vi "SplitPAQsavedPortion.vi"(8 "error in":errorcluster, 9 "split-index":i32, 11 "SaveData in":T1) -> (0 "error out":errorcluster, 2 "SaveData out Day2":T1, 3 "SaveData out Day1":T1)   [LabVIEW 2014, in "DBAL-BIN.lvclass"]
doc: "Split a Database save portion in two halves.\nThe indez input is the point where one day is passed on into another."
uses:
  DBAL-BIN.lvclass
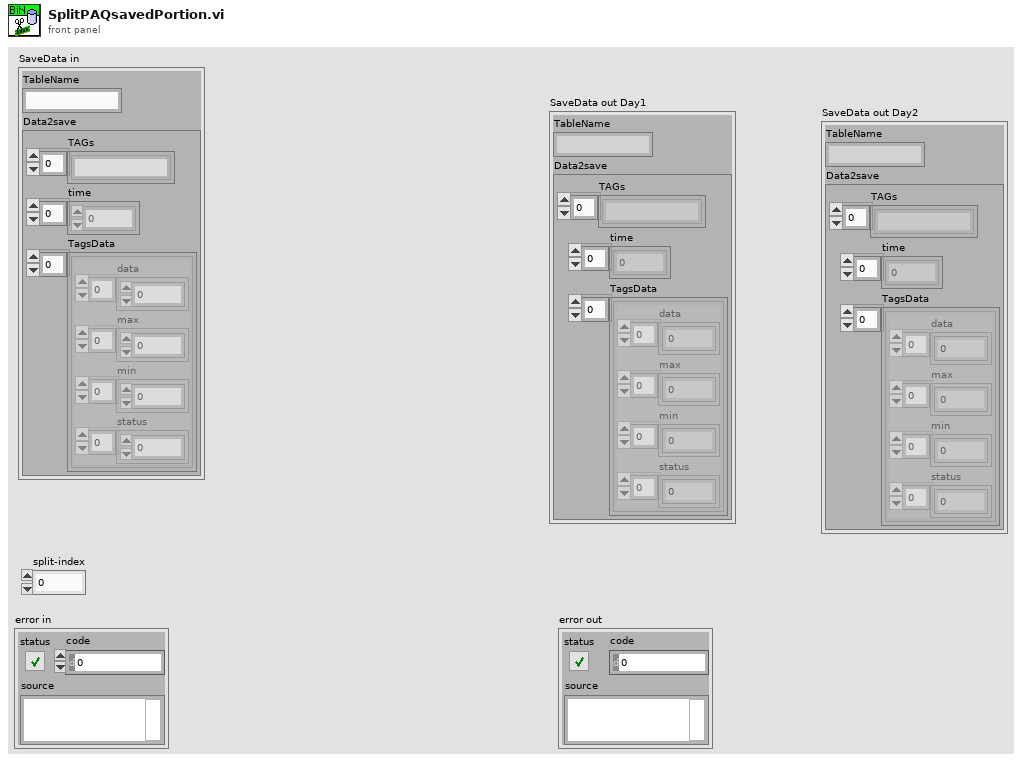
[diagram p1: front panel]
types:
  T1 = cluster{"TableName":string, "Data2save":cluster{"TAGs":string[], "time":dbl[], "TagsData":cluster{"data":dbl[], "max":dbl[], "min":dbl[], "status":u32[]}[]}}
  T2 = cluster{"data":dbl[], "max":dbl[], "min":dbl[], "status":u32[]}[]
  T3 = cluster{"data":dbl[], "max":dbl[], "min":dbl[], "status":u32[]}
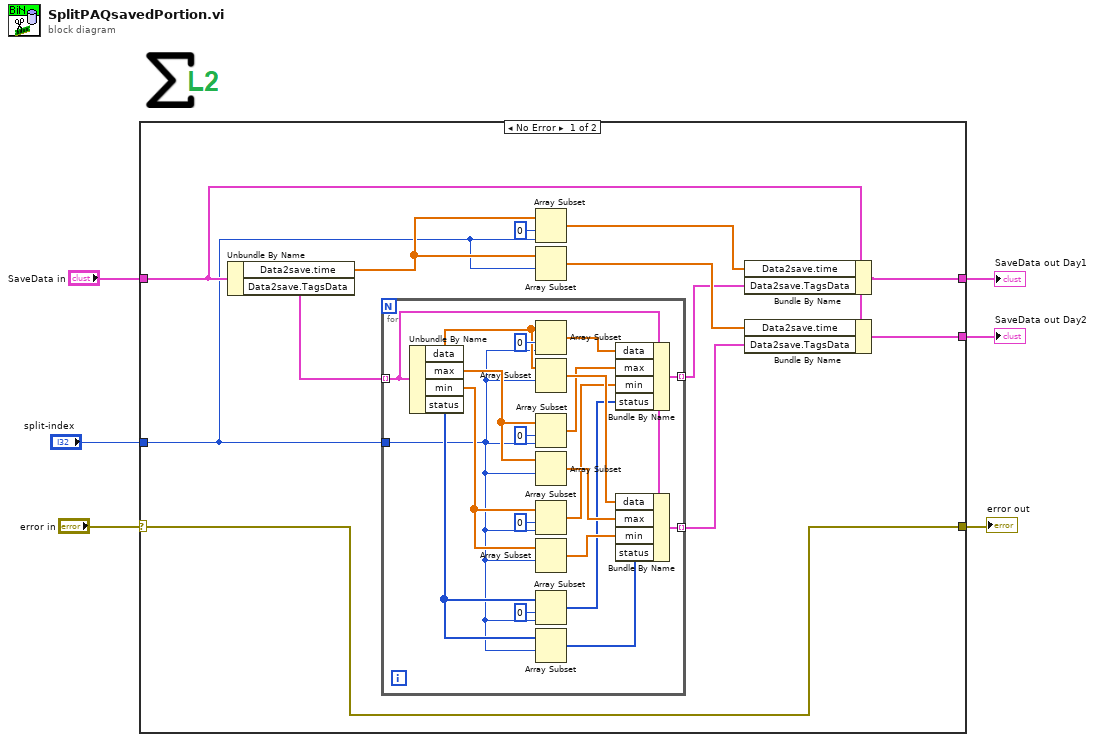
[diagram p0: block diagram]
diagram:
  n1 = case shown="No Error" "error in" {
    selector: "error in" -> [w7 w40]
    tunnel: [w7 w40] -> w6
    tunnel: "SaveData in" -> [w15 w39]
    tunnel: [w17 w39] -> w3
    tunnel: [w16 w39] -> w2
    tunnel: "split-index" -> [w10 _]
    frame No Error {
      n2 = Unbundle By Name(w15) -> ("Data2save.time"=w14:dbl[], "Data2save.TagsData"=w18:T2)
      n3 = for {
        tunnel: w18 -> [w19] mode=indexing
        tunnel: w10 -> [w30]
        tunnel: [w21] -> w9 mode=indexing
        tunnel: [w20] -> w8 mode=indexing
        n4 = Unbundle By Name(w19) -> ("data"=w34:dbl[], "max"=w33:dbl[], "min"=w32:dbl[], "status"=w31:u32[])
        n5 = Array Subset(array=w34, index=0, length=w30) -> (w29:dbl[])
        n6 = Array Subset(array=w34, index=w30) -> (w28:dbl[])  [unwired: 1 in]
        n7 = Array Subset(array=w33, index=0, length=w30) -> (w27:dbl[])
        n8 = Array Subset(array=w33, index=w30) -> (w26:dbl[])  [unwired: 1 in]
        n9 = Array Subset(array=w32, index=0, length=w30) -> (w25:dbl[])
        n10 = Array Subset(array=w32, index=w30) -> (w24:dbl[])  [unwired: 1 in]
        n11 = Array Subset(array=w31, index=0, length=w30) -> (w23:u32[])
        n12 = Array Subset(array=w31, index=w30) -> (w22:u32[])  [unwired: 1 in]
        n13 = Bundle By Name(cluster=w19, "data"=w29, "max"=w27, "min"=w25, "status"=w23) -> (w21:T3)
        n14 = Bundle By Name(cluster=w19, "data"=w28, "max"=w26, "min"=w24, "status"=w22) -> (w20:T3)
      }
      n15 = Array Subset(array=w14, index=0, length=w10) -> (w12:dbl[])
      n16 = Array Subset(array=w14, index=w10) -> (w11:dbl[])  [unwired: 1 in]
      n17 = Bundle By Name(cluster=w15, "Data2save.time"=w12, "Data2save.TagsData"=w9) -> (w17:T1)
      n18 = Bundle By Name(cluster=w15, "Data2save.time"=w11, "Data2save.TagsData"=w8) -> (w16:T1)
    }
    frame Error {
    }
  }
  "error out" <- w6
  "SaveData out Day2" <- w2
  "SaveData out Day1" <- w3
